vi "DCM RT Driver VI.vi"(6 "Device Clock":string, 9 "Device Inputs FIFO":refnum<k33>, 10 "Device Outputs FIFO":refnum<k33>, 11 "Device Reference":T1 format="%.0x") -> ()   [LabVIEW 2016, in "DCM Engine.lvlib"]
uses:
  DCM Engine.lvlib
  <vilib>/NI Veristand/Custom Device API/Custom Device Item Ref.ctl
  <vilib>/Platform/TimedLoop/XDataNode/timing_clust.ctl
  <vilib>/Platform/TimedLoop/XDataNode/nitl_modes.ctl
  <vilib>/Platform/TimedLoop/XDataNode/wakeup.ctl
  <vilib>/Platform/TimedLoop/XDataNode/XDataNode.xnode
  Classes/DCM-NIVS-RT/DCM-NIVS-RT.lvclass
  <vilib>/NI Veristand/Custom Device Tools/Custom Device Utility Library/Custom Device Utility Library.lvlib
  <vilib>/Platform/TimedLoop/XDataNode/XDNodeRunTimeDep.lvlib
  <vilib>/NI VeriStand/Custom Device API/Custom Device API.lvlib
panel:
  in  "Initialization Status Notifier":refnum<notifier>
  in  "Status Notifier":refnum<notifier>
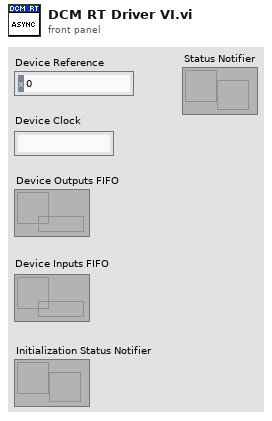
[diagram p1: front panel]
types:
  T1 = typedef "Custom Device API.lvlib/Custom Device Item Ref.ctl" = u64
  T2 = typedef "DCM Shared.lvlib/Compiled Data.ctl" = cluster{"Init":T3, "Cmd Status":T4, "Sys Status":T4, "EPTx RevA":T5, "DCM Core":T8, "DI-A Injection":T18, "DI-B Injection":T18, "DiffIO":T25, "HH Cmd":T28, "DI ADC":T30, "HH ADC":T32, "Digital Signals":T33, "Skip Fire":T34, "Knock":T36, "PBx":T37}
  T3 = typedef "DCM Shared.lvlib/Engine Init Data.ctl" = cluster{"Name":string, "RIO Address":string, "Bitfile Path RT":path, "Username":string, "Password":string, "Cmd CPU":i32, "Cmd Decimation":i32, "Cmd Priority":i32, "Sys CPU":i32, "Sys Decimation":i32, "Sys Priority":i32, "Input FIFO Size":i32, "Output FIFO Size":i32, "Compile Time":dbl}
  T4 = typedef "DCM Shared.lvlib/Engine Status.ctl" = cluster{"FIFO indexes":cluster{"code":i32, "loop duration":i32, "late count":i32}}
  T5 = typedef "DCM Shared.lvlib/EPTx RevA RT Data.ctl" = cluster{"FIFO Indexes":cluster{"Read":cluster{"Sync":i32, "CurrentCAD":i32, "Speed":i32, "Config":i32, "Rcvg Primary":i32, "Stall":i32, "Overflow Error":i32, "Ratio Error":i32, "Pattern Error":i32, "Aux Warning":i32, "Watchdog Error":i32, "Loading":i32}, "Write":cluster{"Reload EPTx":i32, "Sync Enable":i32, "Clear Errors":i32, "Sim Enable":i32, "Sim Speed":i32}}, "Settings":cluster{"EPTxConfigFilename":string, "EPTx Signal Select":cluster{"Primary":T6, "Aux 1":T6, "Aux 2":T6, "Aux 3":T6, "Aux 4":T6}, "FPGAFrequency":sgl, "StallSpeed":sgl, "EPTxFilters":T7, "History":u8}}
  T6 = typedef "DCM-Classes.lvlibp/DCM - FPGA.lvlib/Digital Channel.ctl" = enum8{"Unused", "User OS", "Diff IO 1", "Diff IO 2", "Diff IO 3", "Diff IO 4", "Diff IO 5", "Diff IO 6", "Diff IO 7", "Diff IO 8", "Aux 1", "Aux 2", "Aux 3", "Aux 4", "Aux 5", "Aux 6", "Aux 7", "Aux 8", "Aux 9", "Aux 10", "Aux 11", "Aux 12", "Aux 13", "Aux 14", "Aux 15", "Aux 16"}
  T7 = typedef "DCM-Classes.lvlibp/EPTx - RevA - RT.lvlib/EPTxFilters.ctl" = cluster{"Primary [s]":sgl, "Aux 1 [s]":sgl, "Aux 2 [s]":sgl, "Aux 3 [s]":sgl, "Aux 4 [s]":sgl}
  T8 = typedef "DCM Shared.lvlib/DCM Core.ctl" = cluster{"FIFO Indexes":cluster{"A Run State":i32, "B Run State":i32, "Read":cluster{"Status":T9, "A DI Faults":T10[], "B DI Faults":T10[], "HH Status":T11[]}, "Write":cluster{"A Config":cluster{"PowerSupplyEnable":i32, "InjectEnable":i32, "BoostVoltage":i32}, "B Config":cluster{"PowerSupplyEnable":i32, "InjectEnable":i32, "BoostVoltage":i32}, "HH Config":T12[], "System Settings":cluster{"MPRD":i32, "UserLED1":i32, "UserLED2":i32}, "A Fault Clear":cluster{"1":i32, "2":i32, "3":i32, "4":i32, "5":i32, "6":i32, "7":i32, "8":i32}, "B Fault Clear":cluster{"1":i32, "2":i32, "3":i32, "4":i32, "5":i32, "6":i32, "7":i32, "8":i32}}}, "Settings":cluster{"A Configuration":T13, "B Configuration":T13, "System Settings":T15}}
  T9 = typedef "DCM Shared.lvlib/System State Indexes.ctl" = cluster{"System ADC":cluster{"AI 1 [V]":i32, "AI 2 [V]":i32, "AI 3 [V]":i32, "AI 4 [V]":i32, "AI 5 [V]":i32, "AI 6 [V]":i32, "AI 7 [V]":i32, "AI 8 [V]":i32, "AI 9 [V]":i32, "AI 10 [V]":i32, "AI 11 [V]":i32, "AI 12 [V]":i32, "Temp HH 1-6 [C]":i32, "Temp HH 7-12 [C]":i32, "Temp DI A [C]":i32, "Temp DI Zener A [C]":i32, "Temp DI B [C]":i32, "Temp DI Zener B [C]":i32, "Temp CPU [C]":i32, "Temp Fan Intake [C]":i32, "Temp Secondary A [C]":i32, "Temp Primary A [C]":i32, "Temp Boost B [C]":i32, "Primary Range [V]":i32, "Primary A1A2 [V]":i32, "Primary A3A4 [V]":i32, "Primary B3B4 [V]":i32, "Primary B1B2 [V]":i32, "Secondary A1A2 [V]":i32, "Secondary A3A4 [V]":i32, "Secondary B3B4 [V]":i32, "Secondary B1B2 [V]":i32, "Ext HV A [V]":i32, "Ext HV B [V]":i32, "FET Driver [V]":i32, "Fan [V]":i32, "Battery [V]":i32, "DRVP [V]":i32, "Key [V]":i32, "DI Zener A [V]":i32, "DI Zener B [V]":i32, "Pump Zener A [V]":i32, "Pump Zener B [V]":i32, "MPRD [V]":i32}, "IO Lock":i32, "HH Mode Config Error":i32, "Fan Speed 1 [RPM]":i32, "Fan Speed 2 [RPM]":i32, "Firmware Major Rev":i32, "Firmware Minor Rev":i32, "Internal Fault":i32, "Fault Value":i32}
  T10 = typedef "DCM Shared.lvlib/DI Faults Indexes.ctl" = cluster{"HV Fault":i32, "LV Fault":i32, "LS Fault":i32, "MUX Fault":i32, "Open Warning":i32}
  T11 = typedef "DCM Shared.lvlib/HH Status Indexes.ctl" = cluster{"Current [A]":i32, "Config Error":i32, "Short Fault":i32, "Open Fault":i32, "Period Min [A]":i32, "Period Max [A]":i32, "Period Avg [A]":i32, "On Avg [A]":i32}
  T12 = typedef "DCM Shared.lvlib/HH Config Indexes.ctl" = cluster{"Mode":i32, "IO Lock State":i32, "Phase 1 FP":i32, "Fault Clear":i32, "ISeq":cluster{"Upper [A]":i32, "Lower [A]":i32, "Duration [s]":i32}[]}
  T13 = typedef "DCM - RT.lvclass/Configuration.ctl" = cluster{"Configuration":T14, "Power Supply Enable":bool, "Boost Voltage [V]":sgl, "Inject Enable":bool, "DI Zener Enable":bool, "DI Zener Voltage [V]":sgl, "Pump Zener Enable":bool, "Pump Zener Voltage [V]":sgl, "Boost Clamp [V]":sgl}
  T14 = typedef "DCM - FPGA.lvlib/DI - Bank Configuration.ctl" = enum8{"Solenoid Unipolar 4", "Solenoid Unipolar 7 (Muxed)", "Solenoid Unipolar 8 (Muxed)", "Solenoid Bipolar 2", "Solenoid Bipolar 3 (Muxed)", "Piezo Unipolar 2", "Piezo Unipolar 3 (Muxed)", "Piezo Unipolar 4 (Muxed)", "Piezo Bipolar 2", "Piezo Bipolar 3 (Muxed)"}
  T15 = typedef "DCM - RT.lvclass/System Settings.ctl" = cluster{"MPRD":bool, "IO Lock MPRD Disable":bool, "User LED 1":T16, "User LED 2":T16, "DI HS Fault Filter Time [s]":sgl, "Clamp Fault Filter Time [s]":sgl, "HH Shoot Through Time [s]":sgl, "HH ISeq Dur PS":T17, "HH Open Threshold [A]":sgl}
  T16 = typedef "DCM - RT.lvclass/User LED.ctl" = enum16{"Off", "Yellow", "Green"}
  T17 = typedef "DCM - RT - HH.lvlib/Duration Pre Scale.ctl" = u8
  T18 = typedef "DCM Shared.lvlib/DI.ctl" = cluster{"DI Command Enabled":bool, "Sync Pump Enabled":bool, "FIFO Indexes":cluster{"Write":cluster{"DI Command":T19[], "Pump Command":T19}}, "Settings":T20}
  T19 = typedef "DCM Shared.lvlib/DI Command Indexes.ctl" = cluster{"Mode":i32, "Digital Input":i32, "Default Profile Index":i32, "Cal Freq [Hz]":i32, "Cal Duration [s]":i32, "Cal Increment [s]":i32, "Cal Pulses":i32, "TMP Command Sequence":cluster{"Duration [s]":i32, "Level":i32, "Run/Stop":i32, "Profile Index":i32}[], "EPT TDC Offset [CAD]":i32, "EPT Window Start [DBTDC]":i32, "EPT Window End [DBTDC]":i32, "EPT Angles":cluster{"Enable":i32, "Timing [DBTDC]":i32, "Duration [s]":i32, "Profile Index":i32}[], "EPT Skip Fire":i32, "EPT Skip Index":i32, "EPT Precharge Duration [s]":i32, "EPT Precharge Profile Index":i32}
  T20 = typedef "DCM Shared.lvlib/DI Phase Outputs.ctl" = cluster{"Inj Phase Arrays":T21[][], "Pump Phase Array":T21[], "Pulsewidths [s]":sgl[][]}
  T21 = typedef "DCM - RT - DI.lvlib/Phase.ctl" = cluster{"Drive":T22, "Direction":bool, "Phase Step":T23, "Duration [s]":sgl, "Current High [A]":sgl, "Current Low [A]":sgl, "Voltage High [V]":sgl, "Voltage Low [V]":sgl, "Change":bool, "Current Control":T24, "Period [s]":sgl, "Pulse Width [s]":sgl, "Profile":u8, "Voltage Control":bool}
  T22 = typedef "DCM - FPGA.lvlib/DI - Drive State.ctl" = enum8{"Idle", "HV Current Control", "LV Current Control", "Back Boost", "Piezo Charge", "Piezo Discharge"}
  T23 = typedef "DCM - FPGA - DI.lvlib/Phase Step.ctl" = enum8{"Duration", "First Peak", "End of Cmd", "Branch", "2-Phase Duration"}
  T24 = typedef "DCM - FPGA - DI.lvlib/Control.ctl" = enum8{"Closed Loop", "Fixed Period", "Fixed On Pulse", "Fixed Off Pulse", "Open Loop", "Profile"}
  T25 = typedef "DCM Shared.lvlib/DiffIO.ctl" = cluster{"DiffIO Command Enabled":bool, "FIFO Indexes":cluster{"Read":cluster{"Diff IO Results":T26[], "DiffIOIn":cluster{"1":i32, "2":i32, "3":i32, "4":i32, "5":i32, "6":i32, "7":i32, "8":i32}}, "Write":cluster{"Diff I/O Setup":T27[]}}}
  T26 = typedef "DCM Shared.lvlib/DiffIO Results Indexes.ctl" = cluster{"Capture [DBTDC]":i32, "Capture Error":i32, "Frequency [Hz]":i32, "Duty Cycle [%]":i32, "PWM Stopped":i32}
  T27 = typedef "DCM Shared.lvlib/DiffIO Setup Indexes.ctl" = cluster{"Mode":i32, "Capture Start [DBTDC]":i32, "Capture End [DBTDC]":i32, "Invert":i32, "Frequency [Hz]":i32, "Duty Cycle [%]":i32, "TDC Offset [CAD]":i32, "Window Start [DBTDC]":i32, "Window End [DBTDC]":i32, "Angles":cluster{"Enable":i32, "Location [DBTDC]":i32, "Duration [s]":i32}[], "Skip Fire":i32, "Skip Fire Index":i32}
  T28 = typedef "DCM Shared.lvlib/HH.ctl" = cluster{"HH Command Enabled":bool, "FIFO Indexes":cluster{"Write":T29[]}}
  T29 = typedef "DCM Shared.lvlib/HH Command Indexes.ctl" = cluster{"Mode":i32, "Digital Input":i32, "Polarity":i32, "Frequency [Hz]":i32, "Duty Cycle [%]":i32, "TDC Offset [CAD]":i32, "Window Start [DBTDC]":i32, "Window End [DBTDC]":i32, "Angles":cluster{"Enable":i32, "Location [DBTDC]":i32, "Duration [s]":i32}[], "Skip Fire":i32, "Skip Fire Index":i32}
  T30 = typedef "DCM Shared.lvlib/DI Scope.ctl" = cluster{"FIFO Indexes":cluster{"Write":cluster{"Capture Enable":i32, "Capture Event":i32, "Capture Length":i32, "DI ADC 1 Select":i32, "DI ADC 2 Select":i32, "DI ADC 3 Select":i32, "DI ADC 4 Select":i32}, "Read":cluster{"Capture dt [s]":i32}}, "DI ADC Data":cluster{"Output Array":sgl[][], "New Data":bool}, "Waveform Data":T31[], "Waveform Session":refnum<class "Multiple Waveforms Write (DBL).lvclass">}
  T31 = typedef "Custom Device API.lvlib/Waveform Data Reference.ctl" = i32
  T32 = typedef "DCM Shared.lvlib/HH Scope.ctl" = cluster{"FIFO Indexes":cluster{"Write":cluster{"Capture Enable":i32, "Capture Event":i32, "Capture Length":i32}, "Read":cluster{"Capture dt [s]":i32}}, "HH ADC Data":cluster{"Output Array":sgl[][], "New Data":bool}, "Waveform Data":T31[], "Waveform Session":refnum<class "Multiple Waveforms Write (DBL).lvclass">}
  T33 = typedef "DCM Shared.lvlib/Digital Signals.ctl" = cluster{"FIFO Indexes":cluster{"Write":cluster{"User OS":i32, "User OS Time [s]":i32}}, "Settings":cluster{"Diff IO Filters [s]":sgl[], "Aux In Filters [s]":sgl[], "Serial In 1":T6, "Serial In 2":T6}}
  T34 = typedef "DCM Shared.lvlib/Skip Fire.ctl" = cluster{"Skip Fire Enabled":bool, "FIFO Indexes":cluster{"Write":cluster{"Setup":T35[]}}}
  T35 = typedef "DCM Shared.lvlib/Skip Fire Setup Indexes.ctl" = cluster{"Enable":i32, "Total Cycles":i32, "On Cycles":i32, "TDC Offset [CAD]":i32}
  T36 = typedef "DCM Shared.lvlib/Knock.ctl" = cluster{"Knock Enabled":bool, "FIFO Indexes":cluster{"Read":cluster{"Knock":i32[], "Knock Intensity":i32[]}, "Write":cluster{"Low Cutoff [Hz]":i32, "High Cutoff [Hz]":i32, "Threshold":i32, "Knock Start [CAD]":i32, "Knock End [CAD]":i32, "Reference Start [CAD]":i32, "Reference End [CAD]":i32}}, "Settings":cluster{"Sensor Select":i32[], "Cylinder Offset [CAD]":sgl[]}}
  T37 = typedef "DCM Shared.lvlib/PBx.ctl" = cluster{"PB Version":u8, "PB-01":T38}
  T38 = typedef "DCM Shared.lvlib/PB-01.ctl" = cluster{"FIFO Indexes":cluster{"Write":cluster{"Clear Faults":i32, "ESTTL Setup":T39[], "UEGO Control":cluster{"UEGO1Enable":i32, "UEGO2Enable":i32, "UEGO1Range":i32, "UEGO2Range":i32, "FilterCutoff (Hz)":i32}}, "Read":cluster{"UEGO Sensor Results":cluster{"UEGO1Lambda":i32, "UEGO1Phi":i32, "UEGO1AFRatio":i32, "UEGO1Ip (mA)":i32, "UEGO2Lambda":i32, "UEGO2Phi":i32, "UEGO2AFRatio":i32, "UEGO2Ip (mA)":i32}, "UEGO Temperature (C)":cluster{"UEGO1Temp (C)":i32, "UEGO2Temp (C)":i32, "UEGO1Hot":i32, "UEGO2Hot":i32}, "UEGO Diagnostics":cluster{"UEGO1SensorFault":i32, "UEGO2SensorFault":i32, "UEGO1HeaterFault":i32, "UEGO2HeaterFault":i32, "UEGOFuseStatus":i32, "Battery (V)":i32, "LSUType":i32}}}, "Settings":cluster{"VR-Hall Mode Select":T40[], "VR-Hall Arming Threshold [V]":dbl[], "ESTTL Command Enabled":bool}}
  T39 = typedef "DCM Shared.lvlib/ESTTL Setup Indexes.ctl" = cluster{"Mode":i32, "Polarity":i32, "Frequency [Hz]":i32, "Duty Cycle [%]":i32, "TDC Offset [CAD]":i32, "Window Start [DBTDC]":i32, "Window End [DBTDC]":i32, "Angles":cluster{"Enable":i32, "Location [DBTDC]":i32, "Duration [s]":i32}[], "Skip Fire":i32, "Skip Fire Index":i32}
  T40 = typedef "Vr_Hall_mode_control_revc.ctl" = enum32{"VR Adaptive Arm", "VR Manual Arm", "Hall", "Hall w/ Pull-up"}
  T41 = typedef "XDNodeRunTimeDep.lvlib/timing_clust.ctl" = cluster{"Expected End [f-1]":u64, "Actual End [f-1]":u64, "Finished Late? [f-1]":bool, "Expected End [i-1]":u64, "Actual End [i-1]":u64, "Finished Late? [i-1]":bool, "Expected Start [i]":u64, "Actual Start [i]":u64, "Expected Start [f]":u64, "Actual Start [f]":u64, "Source Name":string, "Structure Name":string, "Period":i64, "Deadline":i64, "Offset":i64, "Start":i64, "Priority":i32, "Timeout":i32, "Mode":T42, "Wakeup Reason":T43, "Error":errorcluster, "Source Type":string, "Secondary Source Type":string, "Global End Time":u64, "Global Start Time":u64, "Frame Duration":u64, "Iteration Duration":u64, "Assigned CPU":i32, "I/O Scan Engine Mode":u32}
  T42 = typedef "XDNodeRunTimeDep.lvlib/nitl_modes.ctl" = enum32{"No Change", "Process missed periods, maintain original phase", "Discard missed periods, maintain original phase", "Process missed periods, ignore original phase", "Discard missed periods, ignore original phase"}
  T43 = typedef "XDNodeRunTimeDep.lvlib/wakeup.ctl" = enum32{"Normal", "Aborted", "Asynchronous wakeup", "Timing source error", "Timed loop error", "Timeout"}
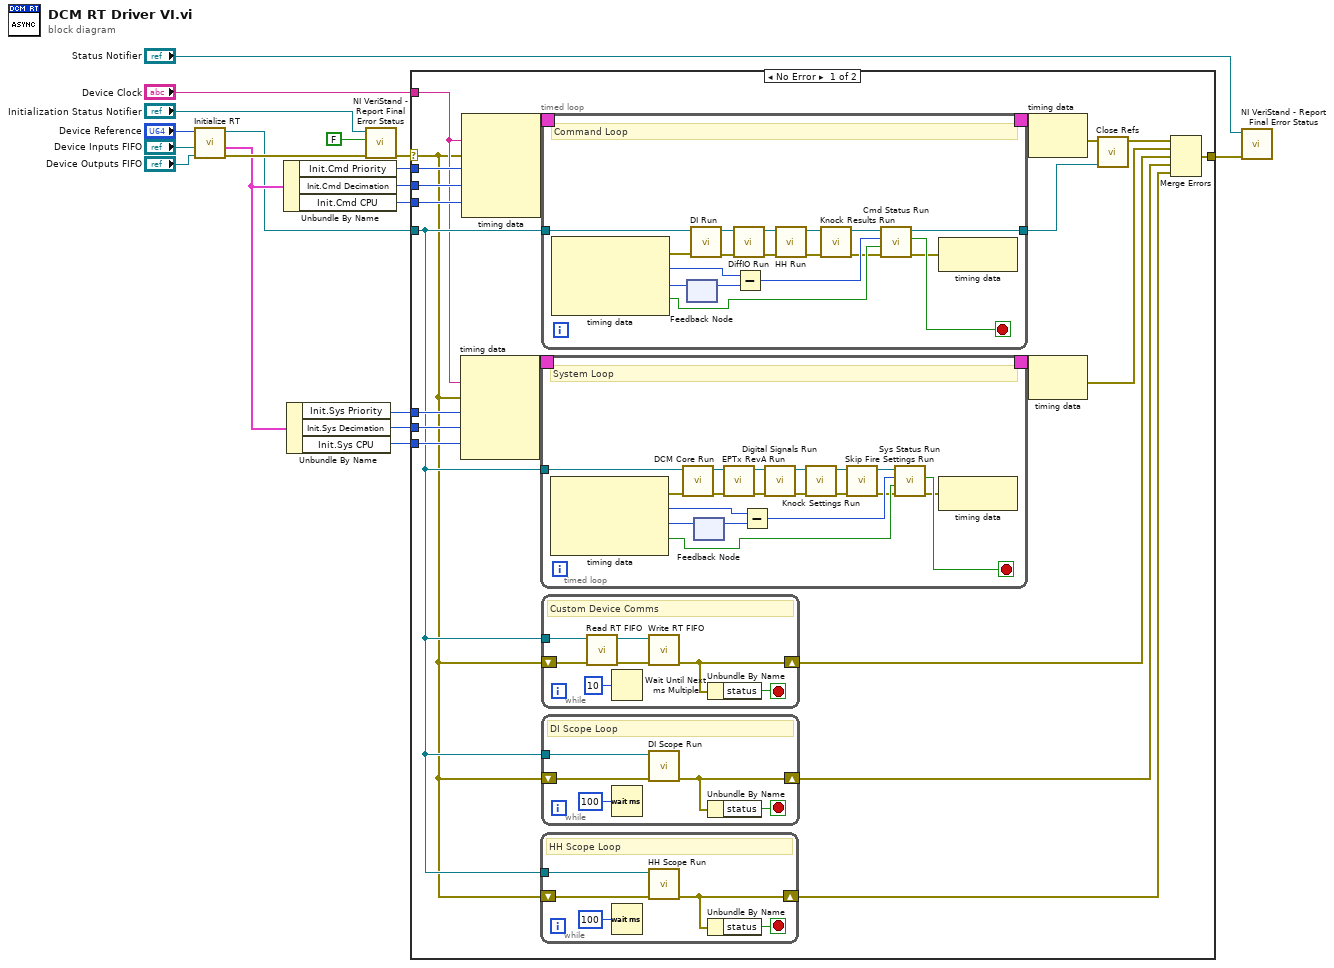
[diagram p0: block diagram]
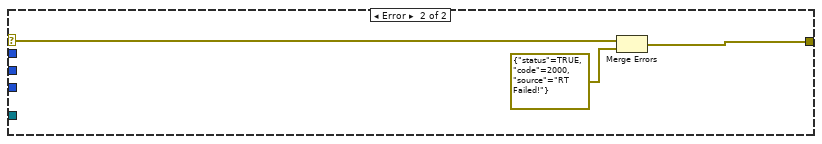
[diagram p2: hidden frame]
diagram:
  n1 = call "Initialize RT.vi"("Device Outputs FIFO"="Device Outputs FIFO", "Device Inputs FIFO"="Device Inputs FIFO", "Device Reference"="Device Reference") -> ("error out"=w9:errorcluster, "Compiled Data"=w2:T2, "DCM-NIVS-RT"=w1:refnum<class "DCM-NIVS-RT.lvclass">)  [unwired: 6 in]
  n2 = Unbundle By Name(w2) -> ("Init.Cmd Priority"=w7:i32, "Init.Cmd Decimation"=w8:i32, "Init.Cmd CPU"=w6:i32)
  n3 = Unbundle By Name(w2) -> ("Init.Sys Priority"=w5:i32, "Init.Sys Decimation"=w4:i32, "Init.Sys CPU"=w3:i32)
  n4 = call <vilib>:"NI VeriStand - Report Final Error Status.vi"("error in (no error)"=w9, "Filter FIFO & Shutdown Errors (T)"=FALSE ("Filter FIFO Errors (T)"), "Status Notifier"="Initialization Status Notifier") -> ("error out"=w11:errorcluster)  [unwired: 8 out]
  n5 = case shown="No Error" w11 {
    selector: w11 -> [w19 w130]
    tunnel: "Device Clock" -> [w20 _]
    tunnel: [w31 w129] -> w14
    tunnel: w8 -> [w37 _]
    tunnel: w7 -> [w36 _]
    tunnel: w6 -> [w35 _]
    tunnel: w1 -> [w22 _]
    tunnel: w5 -> [w28 _]
    tunnel: w4 -> [w27 _]
    tunnel: w3 -> [w26 _]
    frame No Error {
      n6 = node-c288(w20, w19, w28, w27, w26) -> (w30:T41)
      n7 = node-c288 ("Input Node")(w20, w19, w36, w37, w35) -> (w39:T41)
      n8 = timed-loop "SYSTEM LOOP" {
        timing: w30 -> [_]
        timing-out: [_] -> w29
        tunnel: w22 -> [w105]
        stop <- w103 stop-if-true
        # "System Loop"
        n9 = node-c288() -> (w104:errorcluster, w100:i64, w101:i64, w91:bool)  [unwired: 1 in]
        n10 = call "DCM Core Run.vi"("error in"=w104, "RT Data In"=w105) -> ("error out"=w97:errorcluster, "RT Data Out"=w98:refnum<class "DCM-NIVS-RT.lvclass">)  [unwired: 8 in]
        n11 = feedback #1() -> (w102:i64)  [unwired: 1 in]
        n12 = feedback-in #1(w101) -> ()
        n13 = call "EPTx RevA Run.vi"("error in"=w97, "RT Data In"=w98) -> ("error out"=w95:errorcluster, "RT Data Out"=w96:refnum<class "DCM-NIVS-RT.lvclass">)  [unwired: 8 in]
        n14 = Subtract(x=w100, y=w102) -> (x-y=w99:i64)
        n15 = call "Digital Signals Run.vi"("error in"=w95, "RT Data In"=w96) -> ("error out"=w92:errorcluster, "RT Data Out"=w94:refnum<class "DCM-NIVS-RT.lvclass">)  [unwired: 8 in]
        n16 = call "Knock Settings Run.vi"("error in"=w92, "RT Data In"=w94) -> ("error out"=w88:errorcluster, "RT Data Out"=w93:refnum<class "DCM-NIVS-RT.lvclass">)  [unwired: 8 in]
        n17 = call "Skip Fire Settings Run.vi"("error in"=w88, "RT Data In"=w93) -> ("error out"=w87:errorcluster, "RT Data Out"=w89:refnum<class "DCM-NIVS-RT.lvclass">)  [unwired: 8 in]
        n18 = call "Sys Status Run.vi"("error in"=w87, "Finished Late? [i-1]"=w91, "Iteration Duration"=w99, "RT Data In"=w89) -> ("error out"=w90:errorcluster, "Stop"=w103:bool)  [unwired: 5 in, 1 out]
        n19 = node-c288(w90) -> ()  [unwired: 1 out]
      }
      n20 = while {
        shift-right: [w43] -> w21
        shift-left: w19 -> [w40]
        tunnel: w22 -> [w41]
        stop <- w42 stop-if-true
        # "HH Scope Loop"
        n21 = Wait (ms)(milliseconds to wait=u32 100) -> ()  [unwired: 1 out]
        n22 = call "HH Scope Run.vi"("error in"=w40, "RT Data In"=w41) -> ("error out"=w43:errorcluster)  [unwired: 8 in, 1 out]
        n23 = Unbundle By Name(w43) -> ("status"=w42:bool)
      }
      n24 = timed-loop "COMMAND LOOP" {
        timing: w39 -> [_]
        timing-out: [_] -> w38
        tunnel: w22 -> [w65]
        tunnel: [w68] -> w33
        stop <- w69 stop-if-true
        # "Command Loop"
        n25 = node-c288() -> (w66:errorcluster, w63:i64, w64:i64, w60:bool)  [unwired: 1 in]
        n26 = feedback #2() -> (w62:i64)  [unwired: 1 in]
        n27 = feedback-in #2(w64) -> ()
        n28 = call "DI Run.vi"("error in"=w66, "RT Data In"=w65) -> ("error out"=w58:errorcluster, "RT Data Out"=w59:refnum<class "DCM-NIVS-RT.lvclass">)  [unwired: 8 in]
        n29 = call "DiffIO Run.vi"("error in"=w58, "RT Data In"=w59) -> ("error out"=w55:errorcluster, "RT Data Out"=w54:refnum<class "DCM-NIVS-RT.lvclass">)  [unwired: 8 in]
        n30 = Subtract(x=w63, y=w62) -> (x-y=w61:i64)
        n31 = call "HH Run.vi"("error in"=w55, "RT Data In"=w54) -> ("error out"=w52:errorcluster, "RT Data Out"=w53:refnum<class "DCM-NIVS-RT.lvclass">)  [unwired: 8 in]
        n32 = call "Knock Results Run.vi"("error in"=w52, "RT Data In"=w53) -> ("error out"=w56:errorcluster, "RT Data Out"=w57:refnum<class "DCM-NIVS-RT.lvclass">)  [unwired: 8 in]
        n33 = call "Cmd Status Run.vi"("error in"=w56, "Finished Late? [i-1]"=w60, "Iteration Duration"=w61, "RT Data In"=w57) -> ("error out"=w67:errorcluster, "Stop"=w69:bool, "RT Data Out"=w68:refnum<class "DCM-NIVS-RT.lvclass">)  [unwired: 5 in]
        n34 = node-c288(w67) -> ()  [unwired: 1 out]
      }
      n35 = while {
        tunnel: w22 -> [w51]
        shift-right: [w46] -> w23
        shift-left: w19 -> [w48]
        stop <- w47 stop-if-true
        # "Custom Device Comms"
        n36 = call "Read RT FIFO.vi"("error in"=w48, "RT Data In"=w51) -> ("error out"=w49:errorcluster, "RT Data Out"=w50:refnum<class "DCM-NIVS-RT.lvclass">)  [unwired: 8 in]
        n37 = Wait Until Next ms Multiple(millisecond multiple=u32 10) -> ()  [unwired: 1 out]
        n38 = call "Write RT FIFO.vi"("error in"=w49, "RT Data In"=w50) -> ("error out"=w46:errorcluster)  [unwired: 8 in, 1 out]
        n39 = Unbundle By Name(w46) -> ("status"=w47:bool)
      }
      n40 = while {
        shift-right: [w126] -> w24
        shift-left: w19 -> [w123]
        tunnel: w22 -> [w124]
        stop <- w125 stop-if-true
        # "DI Scope Loop"
        n41 = Wait (ms)(milliseconds to wait=u32 100) -> ()  [unwired: 1 out]
        n42 = call "DI Scope Run.vi"("error in"=w123, "RT Data In"=w124) -> ("error out"=w126:errorcluster)  [unwired: 8 in, 1 out]
        n43 = Unbundle By Name(w126) -> ("status"=w125:bool)
      }
      n44 = node-c288(w38) -> (w34:errorcluster)
      n45 = node-c288(w29) -> (w25:errorcluster)
      n46 = call "Close Refs.vi"("RT Data In"=w33, "error in"=w34) -> ("error out"=w32:errorcluster)  [unwired: 9 in]
      n47 = Merge Errors(w32, w25, w23, w24, w21) -> (w31:errorcluster)
    }
    frame Error {
      n48 = Merge Errors(w130, errorcluster {"status"=TRUE, "code"=2000, "source"="RT Failed!"} ("error in")) -> (w129:errorcluster)
    }
  }
  n49 = call <vilib>:"NI VeriStand - Report Final Error Status.vi"("error in (no error)"=w14, "Status Notifier"="Status Notifier") -> ()  [unwired: 1 in, 9 out]
